vi "Write_Config_INI.vi"(7 "section":string, 8 "error in (no error)":errorcluster, 9 "Inputs":string[](array[string]), 10 "Keys":string[](array[string]), 11 "refnum":T1) -> (0 "error out":errorcluster, 3 "refnum 2":T1 caption="引用句柄")   [LabVIEW 2017]
uses:
  <vilib>/Utility/config.llb/Config Data RefNum.ctl
  <vilib>/Utility/config.llb/Write Key (String).vi
  <vilib>/Utility/config.llb/NI_LVConfig.lvlib
panel:
  out "found?":bool caption="已找到？"
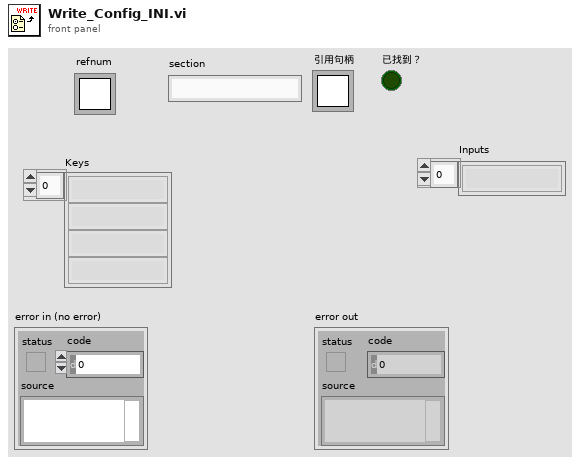
[diagram p1: front panel]
types:
  T1 = typedef "NI_LVConfig.lvlib/Config Data RefNum.ctl" = refnum<k1>
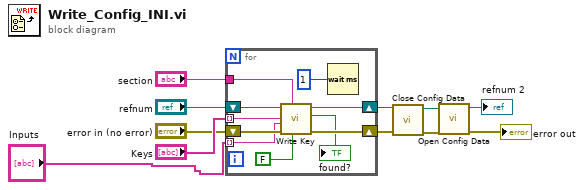
[diagram p0: block diagram]
diagram:
  n1 = for {
    tunnel: "section" -> [w19]
    shift-right: [w20] -> w7
    shift-left: "refnum" -> [w21]
    tunnel: "Keys" -> [w18] mode=indexing
    shift-right: [w16] -> w6
    shift-left: "error in (no error)" -> [w15]
    tunnel: "Inputs" -> [w14] mode=indexing
    n2 = call-poly <vilib>:"Write Key.vi"("write raw string? (F)"=FALSE, "section"=w19, "error in (no error)"=w15, "value"=w14, "key"=w18, "refnum"=w21) -> ("error out"=w16:errorcluster, "found?"=→"found?":bool, "refnum out"=w20:T1)  [unwired: 3 in]
    n3 = Wait (ms)(milliseconds to wait=u32 1) -> ()  [unwired: 1 out]
  }
  n4 = call <vilib>:"Close Config Data.vi"("error in (no error)"=w6, "refnum"=w7) -> ("error out"=w4:errorcluster, "file path"=w5:path)  [unwired: 8 in]
  n5 = call <vilib>:"Open Config Data.vi"("error in (no error)"=w4, "configuration file path"=w5) -> ("error out"=→"error out":errorcluster, "refnum"=→"refnum 2":T1)  [unwired: 7 in, 1 out]
